vi "Digitizer Self Calibration.vi"(11 "error in":errorcluster) -> (15 "error out":errorcluster)   [LabVIEW 2010]
uses:
  <instrlib>/niScope/Controls/niScope self cal option.ctl
  <instrlib>/Tegam4040/Tegam4040.lvlib
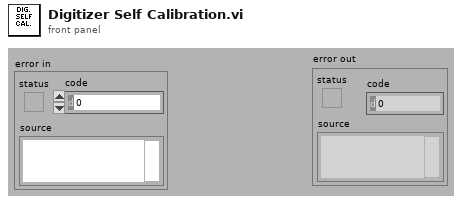
[diagram p1: front panel]
types:
  T1 = typedef "niScope self cal option.ctl" = i32
  T2 = enum16{"Disable Calibration", "Enable Calibration"}
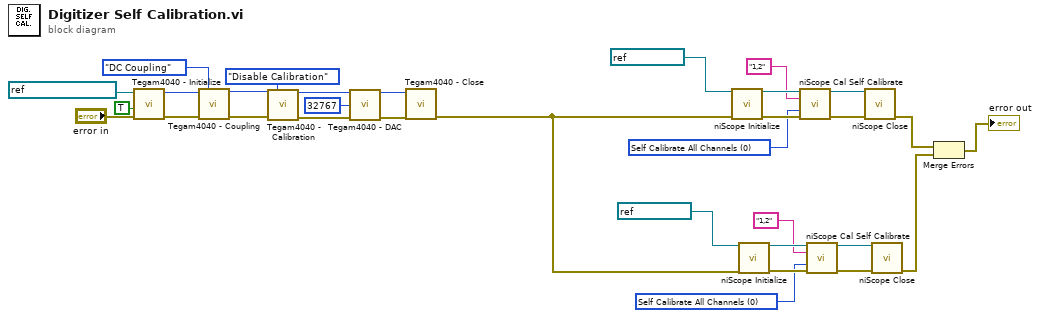
[diagram p0: block diagram]
diagram:
  w5 = T1 0 items=["Self Calibrate All Channels", "Restore External Calibration"] ("Option")
  w12 = T1 0 items=["Self Calibrate All Channels", "Restore External Calibration"] ("Option")
  n1 = call <instrlib>:"Tegam4040 - Initialize.vi"("error in (no error)"="error in", "Reset? (T: Yes)"=TRUE, "VISA Tegam4040"=refnum<visa-resource-name> "PXI4::12::INSTR") -> ("error out"=w23:errorcluster, "Instrument Session Handle"=w24:u32)  [unwired: 7 in]
  n2 = call <instrlib>:"Tegam4040 - Coupling.vi"("Instrument Session Handle In"=w24, "Coupling"=enum16{"DC Coupling", "AC Coupling"}."DC Coupling", "error in (no error)"=w23) -> ("Instrument Session Handle Out (dupl)"=w26:u32, "error out"=w25:errorcluster)  [unwired: 11 in]
  n3 = call <instrlib>:"Tegam4040 - Calibration.vi"("Instrument Session Handle In"=w26, "Calibration"=T2."Disable Calibration", "error in (no error)"=w25) -> ("Instrument Session Handle Out (dupl)"=w30:u32, "error out"=w29:errorcluster)  [unwired: 11 in]
  n4 = call <instrlib>:"Tegam4040 - DAC.vi"("Instrument Session Handle In"=w30, "DAC"=u32 32767, "error in (no error)"=w29) -> ("Instrument Session Handle Out (dupl)"=w20:u32, "error out"=w19:errorcluster)  [unwired: 11 in]
  n5 = call <instrlib>:"Tegam4040 - Close.vi"("error in (no error)"=w19, "Instrument Session Handle"=w20) -> ("error out"=w4:errorcluster)  [unwired: 9 in]
  n6 = call <instrlib>:"niScope Initialize.vi"("resource name"=refnum<k15> "PXI1Slot6", "error in"=w4) -> ("instrument handle"=w17:refnum<k15>, "error out"=w15:errorcluster)  [unwired: 12 in]
  n7 = call <instrlib>:"niScope Initialize.vi"("resource name"=refnum<k15> "PXI1Slot4", "error in"=w4) -> ("instrument handle"=w10:refnum<k15>, "error out"=w8:errorcluster)  [unwired: 12 in]
  n8 = call <instrlib>:"niScope Cal Self Calibrate.vi"("instrument handle"=w17, "channels"="1,2", "Option"=w12, "error in"=w15) -> ("instrument handle out"=w16:refnum<k15>, "error out"=w14:errorcluster)  [unwired: 10 in]
  n9 = call <instrlib>:"niScope Cal Self Calibrate.vi"("instrument handle"=w10, "channels"="1,2", "Option"=w5, "error in"=w8) -> ("instrument handle out"=w9:refnum<k15>, "error out"=w7:errorcluster)  [unwired: 10 in]
  n10 = call <instrlib>:"niScope Close.vi"("instrument handle"=w16, "error in"=w14) -> ("error out"=w3:errorcluster)  [unwired: 13 in]
  n11 = call <instrlib>:"niScope Close.vi"("instrument handle"=w9, "error in"=w7) -> ("error out"=w2:errorcluster)  [unwired: 13 in]
  n12 = Merge Errors(w3, w2) -> (→"error out":errorcluster)
